vi "GetTrigger.vi"(10 "type":string, 11 "triggers":T1[](array[typedef])) -> (1 "found":bool, 2 "trigger":T1)   [LabVIEW 2017, in "DeviceModelHelpers.lvlib"]
uses:
  <vilib>/addons/InsightCM/Utilities/DeviceModelHelpers/DeviceModelHelpers.lvlib
  <vilib>/addons/InsightCM/MessageBus/Base/controls/Trigger.ctl
  <vilib>/addons/InsightCM/MessageBus/Base/controls/Condition.ctl
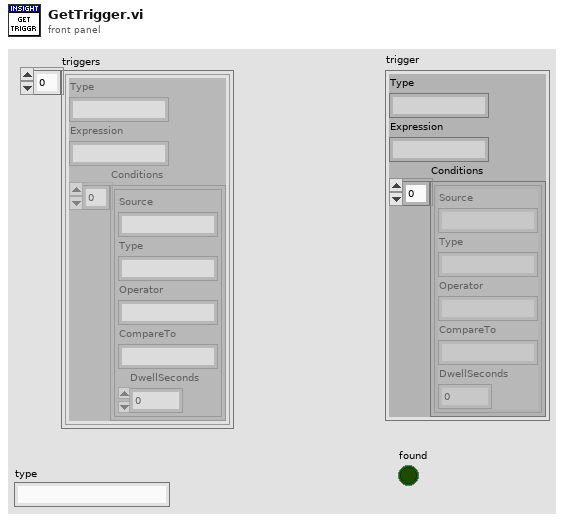
[diagram p1: front panel]
types:
  T1 = typedef "Trigger.ctl" = cluster{"Type":string, "Expression":string, "Conditions":T2[]}
  T2 = typedef "Condition.ctl" = cluster{"Source":string, "Type":string, "Operator":string, "CompareTo":string, "DwellSeconds":dbl}
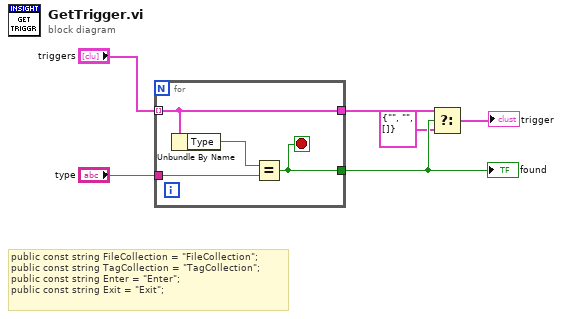
[diagram p0: block diagram]
diagram:
  # "public const string FileCollection = \"FileCollection\";\npublic const string TagCollection = \"TagCollection\";\npublic const string Enter = \"Enter\";\npublic const string Exit = \"Exit\";"
  n1 = for {
    tunnel: "triggers" -> [w8] mode=indexing
    tunnel: "type" -> [w9]
    tunnel: [w8] -> w4
    tunnel: [w7] -> w5
    stop <- w7 stop-if-true
    n2 = Unbundle By Name(w8) -> ("Type"=w10:string)
    n3 = Equal?(x=w10, y=w9) -> (x = y?=w7:bool)
  }
  "found" <- w5
  n4 = Select(t=w4, s=w5, f=T1 {"Type"="", "Expression"="", "Conditions"=[]}) -> (s? t:f=→"trigger":T1)
